vi "Untitled 1.vi"() -> ()   [LabVIEW 2016]
panel:
  in  "stop":bool
  in  "Slide":dbl(slide) scale=-30.0..200.0
  out "Slide 2":dbl(slide) scale=-30.0..200.0
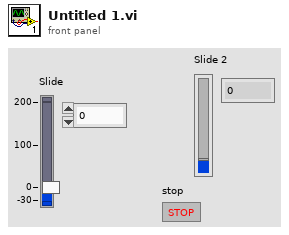
[diagram p1: front panel]
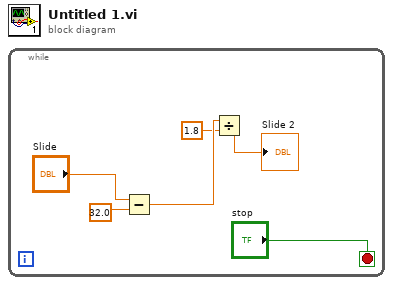
[diagram p0: block diagram]
diagram:
  n1 = while {
    stop <- "stop" stop-if-true
    n2 = Subtract(x="Slide", y=32.0) -> (x-y=w3:dbl)
    n3 = Divide(x=w3, y=1.8) -> (x/y=→"Slide 2":dbl)
  }
